vi "Get Status Channels.vi"(8 "error in":errorcluster, 11 "message or subaddress":T1 format="%.0x") -> (0 "error out":errorcluster, 2 "status channels":T1[](array[typedef]) format="%.0x", 3 "message or subaddress out":T1 format="%.0x", 4 "found?":bool)   [LabVIEW 2020, in "AIM MIL-STD-1553 Scripting.lvlib"]
doc: "Returns the <b>status channels</b> for specified <b>message or subaddress</b>."
uses:
  AIM MIL-STD-1553 Scripting.lvlib
  <vilib>/NI VeriStand/Custom Device API/Custom Device Item Ref.ctl
  Constants.vi
  <vilib>/NI VeriStand/Custom Device Tools/Custom Device Utility Library/NI VeriStand - Search for All Items by GUID.vi
  <vilib>/NI VeriStand/Custom Device Tools/Custom Device Utility Library/Custom Device Utility Library.lvlib
  <vilib>/NI VeriStand/Custom Device API/Custom Device API.lvlib
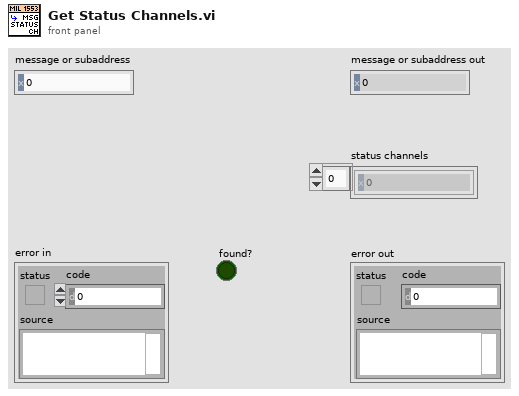
[diagram p1: front panel]
types:
  T1 = typedef "Custom Device API.lvlib/Custom Device Item Ref.ctl" = u64
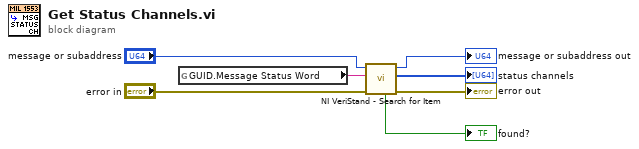
[diagram p0: block diagram]
diagram:
  n1 = global read "Constants.vi" "GUID.Message Status Word"() -> (w6:string)
  n2 = call-poly <vilib>:"NI VeriStand - Search for Item.vi"("error in"="error in", "Item GUID"=w6, "Section Ref in"="message or subaddress") -> ("error out"=→"error out":errorcluster, "Item Refs"=→"status channels":T1[], "Section Ref out"=→"message or subaddress out":T1, "Found"=→"found?":bool)  [unwired: 5 in]
